vi "Servo full.vi"() -> ()   [LabVIEW 2018]
uses:
  <vilib>/myRIO/Instrument Drivers/Onboard IO/PWM/typedefs/PWM Reference.ctl
  <vilib>/myRIO/Common/Instrument Driver Framework/Utilities/typedefs/myRIO Generic Hardware Reference.ctl
  <vilib>/myRIO/Common/Instrument Driver Framework/Utilities/typedefs/Hardware Version Enum.ctl
  <vilib>/myRIO/Common/Instrument Driver Framework/Utilities/typedefs/myRIO v1.0 Reference.ctl
  <vilib>/myRIO/Common/Instrument Driver Framework/Utilities/typedefs/Generic FPGA Reference.ctl
  <vilib>/myRIO/Common/Instrument Driver Framework/myRIO v1.0/PWM/typedefs/PWM Channels Enum.ctl
  <vilib>/myRIO/Instrument Drivers/Onboard IO/PWM/typedefs/PWM Configuration.ctl
  <vilib>/userdefined/High Color/nirio_resource_hc.ctl
  <vilib>/myRIO/Common/Instrument Driver Framework/myRIO v1.0/PWM/vis/myRIO v1.1 Open PWM.vi
  <vilib>/myRIO/Common/Instrument Driver Framework/Utilities/vis/Validate Channels.vi
  <vilib>/myRIO/Common/Instrument Driver Framework/myRIO v1.0/PWM/vis/myRIO v1.0 Reserve PWM.vi
  <vilib>/myRIO/Common/Instrument Driver Framework/myRIO v1.0/UART/vis/myRIO v1.0 Close UART.vi
  <vilib>/myRIO/Common/Instrument Driver Framework/myRIO v1.0/PWM/vis/myRIO v1.0 Build MUX Configuration PWM.vi
  <vilib>/myRIO/Common/Instrument Driver Framework/myRIO v1.0/Resource Manager/vis/myRIO v1.0 Reserve Channel List.vi
  <vilib>/myRIO/Common/Instrument Driver Framework/myRIO v1.0/Resource Manager/vis/myRIO v1.0 Create Configuration List.vi
  <vilib>/myRIO/Common/Instrument Driver Framework/myRIO v1.0/Resource Manager/vis/myRIO v1.0 Reserve Channel.vi
  <vilib>/myRIO/Common/Instrument Driver Framework/myRIO v1.0/Resource Manager/vis/myRIO v1.0 Unreserve Channel.vi
  <vilib>/myRIO/Common/Instrument Driver Framework/myRIO v1.0/Resource Manager/vis/myRIO v1.0 Build Mutex Name.vi
  <vilib>/Utility/VariantDataType/GetNumericInfo.vi
  <vilib>/Utility/error.llb/Error Cluster From Error Code.vi
  <vilib>/myRIO/Common/Instrument Driver Framework/myRIO v1.0/myRIO v1.1 Open.vi
  <vilib>/myRIO/Common/Instrument Driver Framework/Utilities/vis/IO Manager.vi
  <vilib>/myRIO/Common/Instrument Driver Framework/Utilities/vis/Configuration Manager.vi
  <vilib>/myRIO/Common/Instrument Driver Framework/myRIO v1.0/Resource Manager/vis/myRIO v1.0 Configure IO.vi
  <vilib>/myRIO/Common/Instrument Driver Framework/myRIO v1.0/myRIO v1.0 Close.vi
  <vilib>/myRIO/Common/Instrument Driver Framework/myRIO v1.0/PWM/vis/myRIO v1.0 Write PWM.vi
  <vilib>/myRIO/Common/Instrument Driver Framework/Utilities/vis/FPGA Ref Manager.vi
  <vilib>/myRIO/Common/Instrument Driver Framework/myRIO v1.0/myRIO v1.0 Reset FPGA.vi
  <vilib>/myRIO/Common/Instrument Driver Framework/myRIO v1.0/IRQ/vis/myRIO v1.0 IRQ Info FGV.vi
  <vilib>/myRIO/Common/Instrument Driver Framework/myRIO v1.0/IRQ/vis/myRIO v1.0 Timer IRQ Info FGV.vi
  <vilib>/myRIO/Common/Instrument Driver Framework/myRIO v1.0/IRQ/vis/myRIO v1.0 ISR Agent.vi
  <vilib>/myRIO/Instrument Drivers/Onboard IO/PWM/vis/myRIO PWM Open.xnode
  <vilib>/myRIO/Instrument Drivers/Onboard IO/PWM/PWM.lvlib
  <vilib>/myRIO/Instrument Drivers/Utilities/Utilities.lvlib
panel:
  in  "Stop":bool
  in  "Center pixel":dbl format="%#_13g"
  in  "Pixel value":dbl format="%#_13g"
  in  "Center pixel 2":dbl format="%#_13g"
  in  "Pixel value 2":dbl format="%#_13g"
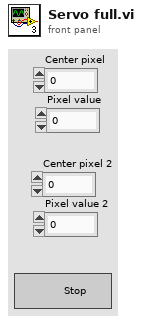
[diagram p1: front panel]
types:
  T1 = typedef "nirio_resource_hc.ctl" = tag
  T2 = typedef "Hardware Version Enum.ctl" = enum16{"Unknown", "myRIO-1900", "myRIO-1950", "roboRIO", "NI ELVIS RIO CM", "ELVIS III"}
  T3 = typedef "PWM.lvlib/PWM Reference.ctl" = cluster{"myRIO Reference":T4, "PWM Channels Enum":T7, "PWM Configuration":T8}
  T4 = typedef "myRIO Generic Hardware Reference.ctl" = cluster{"myRIO Model":T2, "myRIO Hardware Reference":T5}
  T5 = typedef "myRIO v1.0 Reference.ctl" = cluster{"Generic FPGA Reference":T6, "Allow multiple opens":bool}
  T6 = typedef "Generic FPGA Reference.ctl" = refnum<k20>
  T7 = typedef "PWM Channels Enum.ctl" = enum16{"Not Connected", "C/PWM0", "C/PWM1", "A/PWM0", "A/PWM1", "A/PWM2", "A/PWM3", "A/PWM4", "A/PWM5", "A/PWM6", "A/PWM7", "A/PWM8", "A/PWM9", "A/PWM10", "A/PWM11", "A/PWM12", "A/PWM13", "A/PWM14", "A/PWM15", "A/PWM16", "A/PWM17", "A/PWM18", "A/PWM19", "B/PWM0", "B/PWM1", "B/PWM2", "B/PWM3", "B/PWM4", "B/PWM5", "B/PWM6", "B/PWM7", "B/PWM8", "B/PWM9", "B/PWM10", "B/PWM11", "B/PWM12", "B/PWM13", "B/PWM14", "B/PWM15", "B/PWM16", "B/PWM17", "B/PWM18", "B/PWM19", "PWM/PWM0", "PWM/PWM1", "PWM/PWM2", "PWM/PWM3", "PWM/PWM4", "PWM/PWM5", "PWM/PWM6", "PWM/PWM7", "PWM/PWM8", "PWM/PWM9"}
  T8 = typedef "PWM.lvlib/PWM Configuration.ctl" = cluster{"Frequency":dbl, "Duty Cycle":dbl}
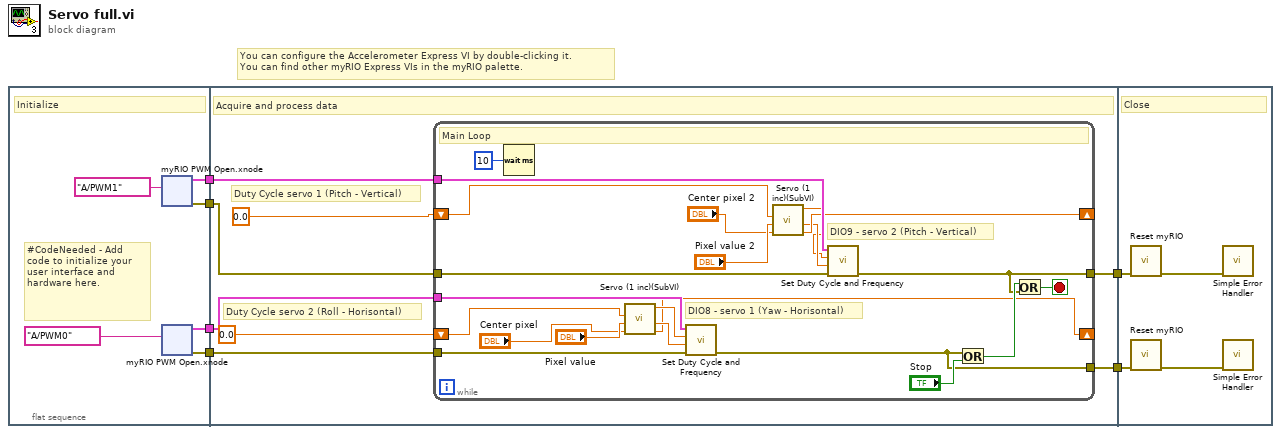
[diagram p0: block diagram]
diagram:
  # "You can configure the Accelerometer Express VI by double-clicking it.\nYou can find other myRIO Express VIs in the myRIO palette."
  n1 = flat-sequence {
    tunnel: [w12] -> w6
    tunnel: [w11] -> w5
    tunnel: [w8] -> w4
    tunnel: [w7] -> w3
    tunnel: [w50] -> w2
    tunnel: w6 -> [w52]
    tunnel: w5 -> [w51]
    tunnel: w4 -> [w49]
    tunnel: w3 -> [w48]
    tunnel: [w47] -> w1
    tunnel: w2 -> [w78]
    tunnel: w1 -> [w75]
    frame #0 {
      # "#CodeNeeded - Add code to initialize your user interface and hardware here."
      # "Initialize"
      n2 = xnode "myRIO PWM Open.xnode"("Channel Name"=tag "A/PWM1") -> ("error out"=w7:errorcluster, "PWM Ref Out"=w8:T3)  [unwired: 2 in]
      n3 = xnode "myRIO PWM Open.xnode"("Channel Name"=tag "A/PWM0") -> ("error out"=w11:errorcluster, "PWM Ref Out"=w12:T3)  [unwired: 2 in]
    }
    frame #1 {
      # "Duty Cycle servo 2 (Roll - Horisontal)"
      # "Duty Cycle servo 1 (Pitch - Vertical)"
      # "Acquire and process data"
      n4 = while {
        tunnel: w52 -> [w73]
        tunnel: w51 -> [w72]
        tunnel: [w71] -> w50
        tunnel: w49 -> [w70]
        tunnel: w48 -> [w69]
        tunnel: [w67] -> w47
        shift-right: [w60] -> _
        shift-left: 0.0 ("Duty Cycle servo 1 (Yaw - Horisontal)") -> [w63]
        shift-right: [w57] -> _
        shift-left: 0.0 ("Duty Cycle servo 1 (Yaw - Horisontal)") -> [w59]
        stop <- w66 stop-if-true
        # "DIO9 - servo 2 (Pitch - Vertical)"
        # "DIO8 - servo 1 (Yaw - Horisontal)"
        # "Main Loop"
        n5 = Wait (ms)(milliseconds to wait=u32 10) -> ()  [unwired: 1 out]
        n6 = call "Servo (1 inc)(SubVI).vi"("Center pixel"="Center pixel", "Pixel value"="Pixel value", "Position."=w63) -> ("Position 2"=w60:dbl, "freq [Hz]"=w61:dbl, "Duty"=w62:dbl)  [unwired: 4 in, 2 out]
        n7 = call <vilib>:"Set Duty Cycle and Frequency.vi"("error in (no error)"=w72, "Frequency [Hz]"=w61, "Duty Cycle"=w62, "PWM Ref In"=w73) -> ("error out"=w71:errorcluster)  [unwired: 5 in, 1 out]
        n8 = call "Servo (1 inc)(SubVI).vi"("Center pixel"="Center pixel 2", "Pixel value"="Pixel value 2", "Position."=w59) -> ("Position 2"=w57:dbl, "freq [Hz]"=w56:dbl, "Duty"=w55:dbl)  [unwired: 4 in, 2 out]
        n9 = call <vilib>:"Set Duty Cycle and Frequency.vi"("error in (no error)"=w69, "Frequency [Hz]"=w56, "Duty Cycle"=w55, "PWM Ref In"=w70) -> ("error out"=w67:errorcluster)  [unwired: 5 in, 1 out]
        n10 = Or(x=w71, y="Stop") -> (x .or. y?=w68:bool)
        n11 = Or(x=w68, y=w67) -> (x .or. y?=w66:bool)
      }
    }
    frame #2 {
      # "Close"
      n12 = call <vilib>:"Reset myRIO.vi"("error in (no error)"=w75) -> ("error out"=w76:errorcluster)  [unwired: 10 in]
      n13 = call <vilib>:"Reset myRIO.vi"("error in (no error)"=w78) -> ("error out"=w77:errorcluster)  [unwired: 10 in]
      n14 = call <vilib>:"Simple Error Handler.vi"("error in (no error)"=w76) -> ()  [unwired: 4 in, 5 out]
      n15 = call <vilib>:"Simple Error Handler.vi"("error in (no error)"=w77) -> ()  [unwired: 4 in, 5 out]
    }
  }
